vi "Request.vi"(11 "WebSocket Client in":refnum<class "WebSocket Client.lvclass">) -> (2 "Request":refnum<class "Request.lvclass">, 3 "WebSocket Client out":refnum<class "WebSocket Client.lvclass">)   [LabVIEW 2020, in "HTTP Server.lvlib" / "WebSocket Client.lvclass"]
uses:
  WebSocket Client.lvclass
  WebSocket Client.lvclass/WebSocket Client.ctl
  lv-http-util/HTTP Utils/Request/Request.lvclass
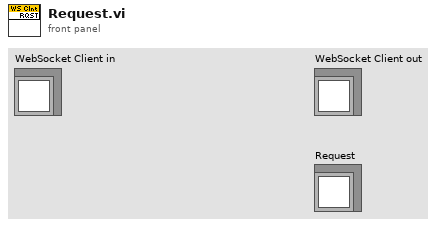
[diagram p1: front panel]
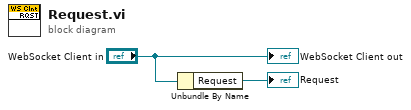
[diagram p0: block diagram]
diagram:
  n1 = Unbundle By Name("WebSocket Client in") -> ("Request"=→"Request":refnum<class "Request.lvclass">)
  "WebSocket Client out" <- "WebSocket Client in"
